vi "20170516-lecture4-2 prof InvokeNodeToolbarControl.vi"() -> ()   [LabVIEW 2014]
panel:
  in  "Export plot to clipboard":bool
  out "Waveform Chart":dbl(graph)
  in  "Tool Bar:Visible":bool
  in  "stop":bool
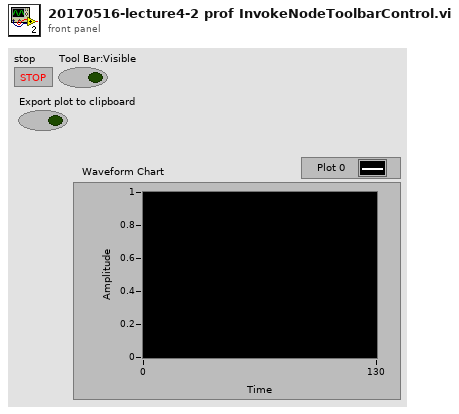
[diagram p1: front panel]
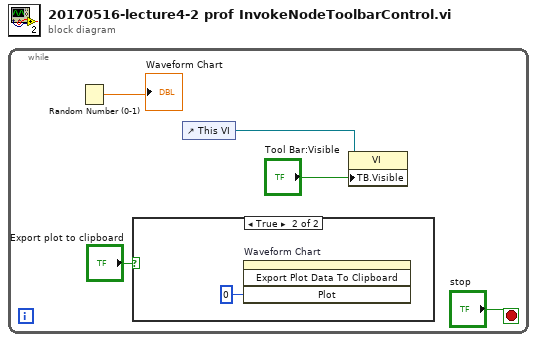
[diagram p0: block diagram]
diagram:
  n1 = while {
    stop <- "stop" stop-if-true
    n2 = Random Number (0-1)() -> (number: 0 to 1=→"Waveform Chart":dbl)
    n3 = case shown="True" "Export plot to clipboard" {
      frame False {
      }
      frame True {
        n4 = invoke on="Waveform Chart" class="WFChart (strict)" method="Export Plot Data To Clipboard"("Plot"=0) -> ()  [unwired: 3 in, 4 out]
      }
    }
    n5 = control-ref of="This VI"() -> (w4:refnum<vi>)
    n6 = property class="VI"(reference=w4, "TB.Visible"="Tool Bar:Visible") -> ()  [unwired: 1 in, 2 out]
  }
